vi "Load Plugin Management Core.vi"(11 "CIFPluginManager in":refnum<class "CIFPluginManager.lvclass">) -> (0 "error out":errorcluster)   [LabVIEW 2021, in "CIFPluginManager.lvclass"]
uses:
  CIFPluginManager.lvclass
  CIFPluginManager.lvclass/CIFPluginManager.ctl
  gRPC/CIF_Manager_server/RPC Service/Manager/Manager.lvclass
  C:/Program Files/National Instruments/LabVIEW 2021/vi.lib/gRPC/LabVIEW gRPC Servicer/ServiceBase/ServiceBase.lvclass
  gRPC/CIF_Manager_server/RPC Service/Manager/Manager.lvclass/Manager.ctl
  gRPC/CIF_Manager_server/RPC Messages/cif_manager_LoadPluginResponse.ctl
  gRPC/CIF_Manager_server/RPC Messages/cif_common_Status.ctl
  typedef/Plugin Load Command.ctl
  typedef/Loader Type.ctl
  CIFCore/Common/Typedef/Errors.ctl
  <vilib>/Utility/miscctls.llb/LVMapReplaceAction.ctl
  typedef/Loader Load Command.ctl
  gRPC/CIF_Manager_server/RPC Messages/cif_manager_AbortPluginResponse.ctl
  gRPC/CIF_Manager_server/RPC Messages/cif_manager_AbortAllPluginsResponse.ctl
  gRPC/CIF_Manager_server/RPC Messages/Get cif_manager_LoadPluginRequest.vi
  gRPC/CIF_Manager_server/RPC Messages/Set cif_manager_LoadPluginResponse.vi
  <vilib>/CIF Foundation/CIF Utilities/Errors/Append Error Location.vi
  gRPC/CIF_Manager_server/RPC Messages/Get cif_manager_AbortPluginRequest.vi
  gRPC/CIF_Manager_server/RPC Messages/Set cif_manager_AbortPluginResponse.vi
  gRPC/CIF_Manager_server/RPC Messages/Get cif_manager_AbortAllPluginsRequest.vi
  gRPC/CIF_Manager_server/RPC Messages/Set cif_manager_AbortAllPluginsResponse.vi
  gRPC/CIF_Manager_server/RPC Messages/Get cif_manager_LoadPluginRequest.vi/2ed25e12-861d-4677-8ead-ace2906b2041.vi
  gRPC/CIF_Manager_server/RPC Messages/FlatToRichcif_manager_LoadPluginRequest.vi
  gRPC/CIF_Manager_server/RPC Messages/Set cif_manager_LoadPluginResponse.vi/dcc74a39-081a-4bdd-860b-8ed792803c96.vi
  gRPC/CIF_Manager_server/RPC Messages/RichToFlatcif_manager_LoadPluginResponse.vi
  gRPC/CIF_Manager_server/RPC Messages/Get cif_manager_AbortPluginRequest.vi/2ed25e12-861d-4677-8ead-ace2906b2041.vi
  gRPC/CIF_Manager_server/RPC Messages/FlatToRichcif_manager_AbortPluginRequest.vi
  gRPC/CIF_Manager_server/RPC Messages/Set cif_manager_AbortPluginResponse.vi/dcc74a39-081a-4bdd-860b-8ed792803c96.vi
  gRPC/CIF_Manager_server/RPC Messages/RichToFlatcif_manager_AbortPluginResponse.vi
  gRPC/CIF_Manager_server/RPC Messages/Get cif_manager_AbortAllPluginsRequest.vi/2ed25e12-861d-4677-8ead-ace2906b2041.vi
  gRPC/CIF_Manager_server/RPC Messages/FlatToRichcif_manager_AbortAllPluginsRequest.vi
  gRPC/CIF_Manager_server/RPC Messages/Set cif_manager_AbortAllPluginsResponse.vi/dcc74a39-081a-4bdd-860b-8ed792803c96.vi
  gRPC/CIF_Manager_server/RPC Messages/RichToFlatcif_manager_AbortAllPluginsResponse.vi
  <vilib>/gRPC/LabVIEW gRPC Library/Shared/TranslateGrpcError.vi
  gRPC/CIF_Manager_server/RPC Messages/RichToFlatcif_common_Status.vi
  <vilib>/gRPC/LabVIEW gRPC Library/Server API/Server/Get Server DLL Path.vi
  <vilib>/Utility/error.llb/Error Cluster From Error Code.vi
  <vilib>/string/Create NI GUID.vi
  <vilib>/gRPC/LabVIEW gRPC Library/Server API/Message Requests/Complete Call.vi
  CIFUtilities/CIFLogs/CIFLogs.lvlib
  CIFCore/Common/CIFCoreCommon.lvlib
  CIFCore/Grpc/CIFCoreWrapper/CIFCoreWrapper.lvlib
  <vilib>/CIF Foundation/CIF Utilities/Time/Time_CIF_U.lvlib
  gRPC/CIF_Manager_Client_Wrapper/CIFManagerClientWrapper.lvlib
  CIFPluginLoader/gRPC/CIF_Plugin_Loader_Client_Wrapper/CIFPluginLoaderClientWrapper.lvlib
  gRPC/CIF_Manager_server/CIF_Manager_server.lvlib
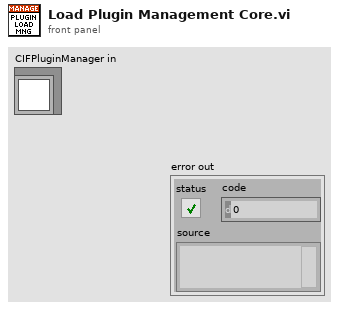
[diagram p1: front panel]
types:
  T1 = typedef "CIF_Manager_server.lvlib/Manager.lvclass/Server gRPC UEs.ctl" = cluster{"Manager LoadPlugin gRPC UE":refnum<user-event>, "Manager RegisterPlugin gRPC UE":refnum<user-event>, "Manager UnregisterPlugin gRPC UE":refnum<user-event>, "Manager QueryPluginTypes gRPC UE":refnum<user-event>, "Manager AbortPlugin gRPC UE":refnum<user-event>, "Manager UnloadAllPlugins gRPC UE":refnum<user-event>, "Manager Destroy gRPC UE":refnum<user-event>, "Manager Ping gRPC UE":refnum<user-event>, "Manager QueryErrors gRPC UE":refnum<user-event>, "Manager QueryConfig gRPC UE":refnum<user-event>, "Manager QueryInfo gRPC UE":refnum<user-event>, "Manager ResetErrorIndex gRPC UE":refnum<user-event>, "Manager ResetConfigIndex gRPC UE":refnum<user-event>, "Manager ResetInfoIndex gRPC UE":refnum<user-event>, "Manager QueryPluginInfo gRPC UE":refnum<user-event>, "Manager QueryPlugin gRPC UE":refnum<user-event>, "Manager QuerySystemStatus gRPC UE":refnum<user-event>, "Manager UpdateClock gRPC UE":refnum<user-event>, "Manager CreateOrch gRPC UE":refnum<user-event>, "Manager QueryClockStatus gRPC UE":refnum<user-event>, "Manager QueryAllChannels gRPC UE":refnum<user-event>, "Manager RegisterPluginLoader gRPC UE":refnum<user-event>, "Manager UnregisterPluginLoader gRPC UE":refnum<user-event>, "Manager CreatePluginLoader gRPC UE":refnum<user-event>, "Manager DestroyPluginLoader gRPC UE":refnum<user-event>, "Manager QueryPluginLoaders gRPC UE":refnum<user-event>}
  T2 = typedef "CIF_Manager_server.lvlib/cif_manager_LoadPluginResponse.ctl" = cluster{"status":T3}
  T3 = typedef "CIF_Manager_server.lvlib/cif_common_Status.ctl" = cluster{"code":i32, "message":string}
  T4 = typedef "CIFPluginManager.lvclass/Plugin Load Command.ctl" = cluster{"Plugin Name":string, "Plugin Path":string, "Loader Name":string, "Loader Type":T5}
  T5 = typedef "CIFPluginManager.lvclass/Loader Type.ctl" = enum16{"LabVIEW"}
  T6 = typedef "CIFCoreCommon.lvlib/Errors.ctl" = enum16{"Invalid Clock ID", "Long Sleep", "gRPC Server Not Found", "Config Parse", "Timestamp Wrap", "Delayed Execution", "Duplicate Channel", "Missing Channel", "Incorrect Type", "Flatten Error", "Unflatten Data", "Unique Name", "Plugin Not Found", "Plugin Type Not Found", "Plugin Version Not Found", "Manager Not Found", "Numerical Issue", "Time Jump", "Clock ID Match", "Channel Length", "Plugin Connection", "gRPC Server Connection", "PPL Name Match", "Build", "Config Log Parse", "Plugin Load", "UI Subpanel Load", "Python Name", "Invalid Name", "Unable to Change Ch Buffer", "Failed Kill", "Failed SysExec", "Function Not Implemented", "Load Timeout"}
  T7 = typedef "LVMapReplaceAction.ctl" = enum32{"Modify Entry only if found", "Add or Modify Entry", "Delete Entry"}
  T8 = typedef "CIFPluginManager.lvclass/Loader Load Command.ctl" = cluster{"Loader Type":T5, "Loader Name":string}
  T9 = typedef "CIF_Manager_server.lvlib/cif_manager_AbortPluginResponse.ctl" = cluster{"status":T3}
  T10 = typedef "CIF_Manager_server.lvlib/cif_manager_AbortAllPluginsResponse.ctl" = cluster{"status":T3}
  T11 = typedef "CIFPluginManager.lvclass/Plugin Management Data Map.ctl" = map{string, T12}
  T12 = typedef "CIFPluginManager.lvclass/Plugin Management Data.ctl" = cluster{"Unique Name":string, "Plugin Type":string, "gRPC Port":i32, "gRPC ID":T13, "Loader Type":T5, "Loader":string, "Version":T14, "Load Timestamp":i64, "Unload Timestamp":i64, "Unloading":bool, "Ready for removal":bool, "status":T15, "channels":T24}
  T13 = typedef "grpc-lvsupport-release.lvlib/grpcId.ctl" = u64
  T14 = typedef "CIFCoreCommon.lvlib/Version.ctl" = cluster{"Major":i32, "Minor":i32, "Fix":i32, "Build":i32}
  T15 = typedef "CIF_Manager_server.lvlib/cif_management_common_PluginStatusData.ctl" = cluster{"state":T16, "timing_statistics":T17, "fifo_statistics":T19, "error":T20, "monitor_doubles":T21, "monitor_u64s":T22, "monitor_i64s":T23}
  T16 = typedef "CIF_Manager_server.lvlib/cif_management_common_PluginStatusData_PluginState.ctl" = enum32{"PLUGINSTATE_UNKNOWN", "PLUGINSTATE_CREATING", "PLUGINSTATE_LISTENING", "PLUGINSTATE_RUNNING", "PLUGINSTATE_CLEANINGUP", "PLUGINSTATE_DESTROYING"}
  T17 = typedef "CIF_Manager_server.lvlib/cif_management_common_TimingStatistics.ctl" = cluster{"period":T18, "wake_error":T18, "execute":T18, "housekeep":T18, "idle":T18, "cleanup":T18, "custom_1":T18, "custom_2":T18}
  T18 = typedef "CIF_Manager_server.lvlib/cif_common_TimingStats.ctl" = cluster{"max":i64, "min":i64, "avg":dbl}
  T19 = typedef "CIF_Manager_server.lvlib/cif_management_common_FifoStatistics.ctl" = cluster{"from_t0":T18, "from_previous_plugin":T18, "output_error":T18}
  T20 = typedef "CIF_Manager_server.lvlib/cif_management_common_Error.ctl" = cluster{"status":bool, "code":i32}
  T21 = typedef "CIF_Manager_server.lvlib/cif_management_common_MonitorDoubles.ctl" = cluster{"double_1":dbl, "double_2":dbl, "double_3":dbl, "double_4":dbl}
  T22 = typedef "CIF_Manager_server.lvlib/cif_management_common_MonitorU64.ctl" = cluster{"u64_1":u64, "u64_2":u64, "u64_3":u64, "u64_4":u64}
  T23 = typedef "CIF_Manager_server.lvlib/cif_management_common_MonitorI64.ctl" = cluster{"i64_1":i64, "i64_2":i64, "i64_3":i64, "i64_4":i64}
  T24 = typedef "CIF_Manager_server.lvlib/cif_management_common_Channels.ctl" = cluster{"channels":T25[]}
  T25 = typedef "CIF_Manager_server.lvlib/cif_management_common_Channel.ctl" = cluster{"name":string, "direction":T26, "type":string, "custom_config":u8[], "connected":bool, "connected_name":string, "forced":bool, "channel_pattern":T27}
  T26 = typedef "CIF_Manager_server.lvlib/cif_management_common_ChannelDirection.ctl" = enum32{"CHANNELDIRECTION_UNKNOWN", "CHANNELDIRECTION_PUBLISHER", "CHANNELDIRECTION_SUBSCRIBER"}
  T27 = typedef "CIF_Manager_server.lvlib/cif_management_common_ChannelPattern.ctl" = enum32{"CHANNELPATTERN_UNKNOWN", "CHANNELPATTERN_TAG", "CHANNELPATTERN_FIFO", "CHANNELPATTERN_MULTIFIFO", "CHANNELPATTERN_BACKPRESSUREFIFO"}
  T28 = typedef "CIF_Manager_server.lvlib/cif_manager_LoadPluginRequest.ctl" = cluster{"plugin_type":string, "plugin_name":string, "version":string, "loader_process":string}
  T29 = typedef "CIFPluginManager.lvclass/Discovered Plugin.ctl" = cluster{"Filename":string, "Plugin Type":string, "Qualified name":string, "Version":T14, "Plugin Metadata":T30, "Loader Type":T5, "File Path":string, "Relative Path":string[]}
  T30 = typedef "CIFPluginManager.lvclass/Plugin Metadata.ctl" = cluster{"Description":string, "History":string, "Author":string}
  T31 = typedef "CIF_Manager_client.lvlib/cif_common_Status.ctl" = cluster{"code":i32, "message":string}
  T32 = typedef "CIFPluginManager.lvclass/Loader Map.ctl" = map{string, T33}
  T33 = typedef "CIFPluginManager.lvclass/Loaders.ctl" = cluster{"Loader Type":T5, "grpc_port":i32, "pid":u32, "gRPC ID":T13, "Load Timestamp":i64, "Unloading":bool, "Ready for removal":bool, "Unload Timestamp":i64}
  T34 = typedef "CIF_Manager_server.lvlib/cif_manager_AbortPluginRequest.ctl" = cluster{"plugin_name":string}
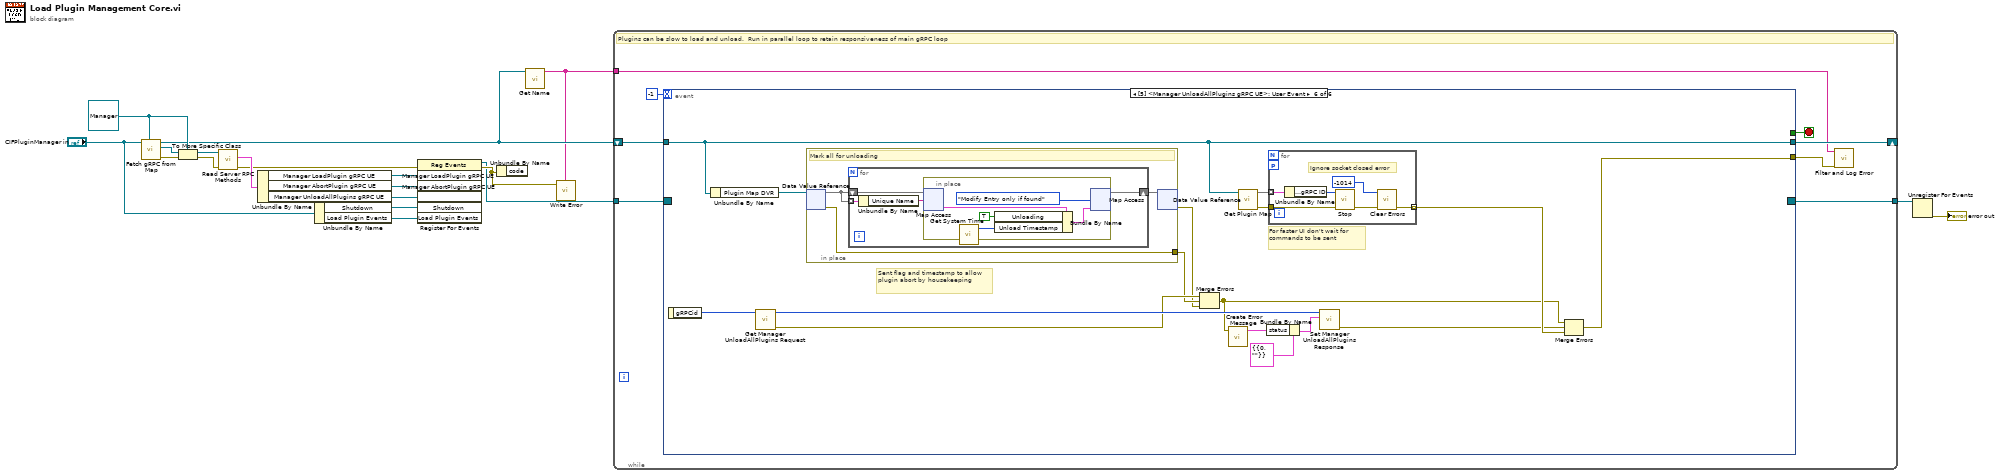
[diagram p0: block diagram]
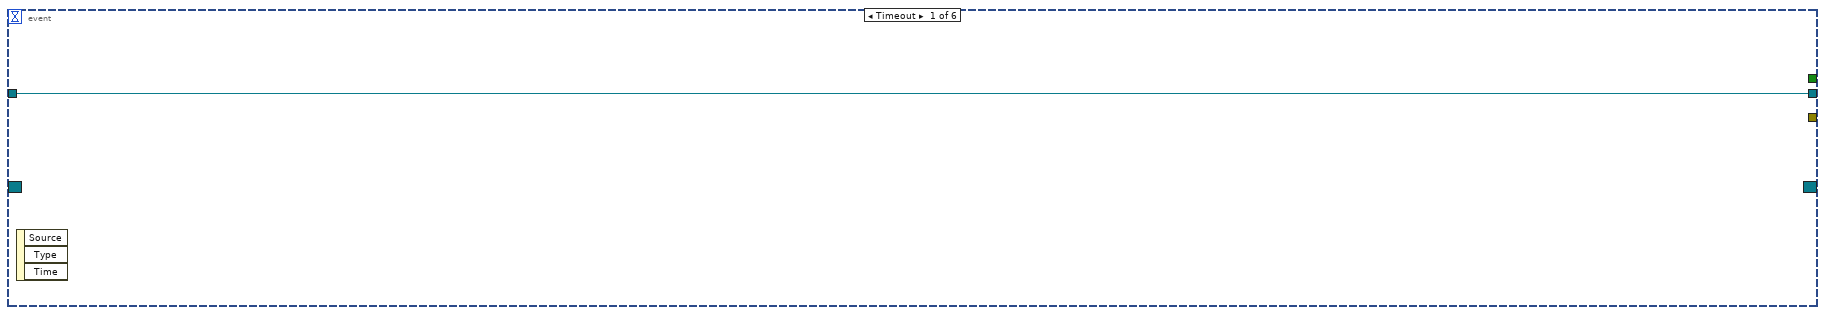
[diagram p2: hidden frame]
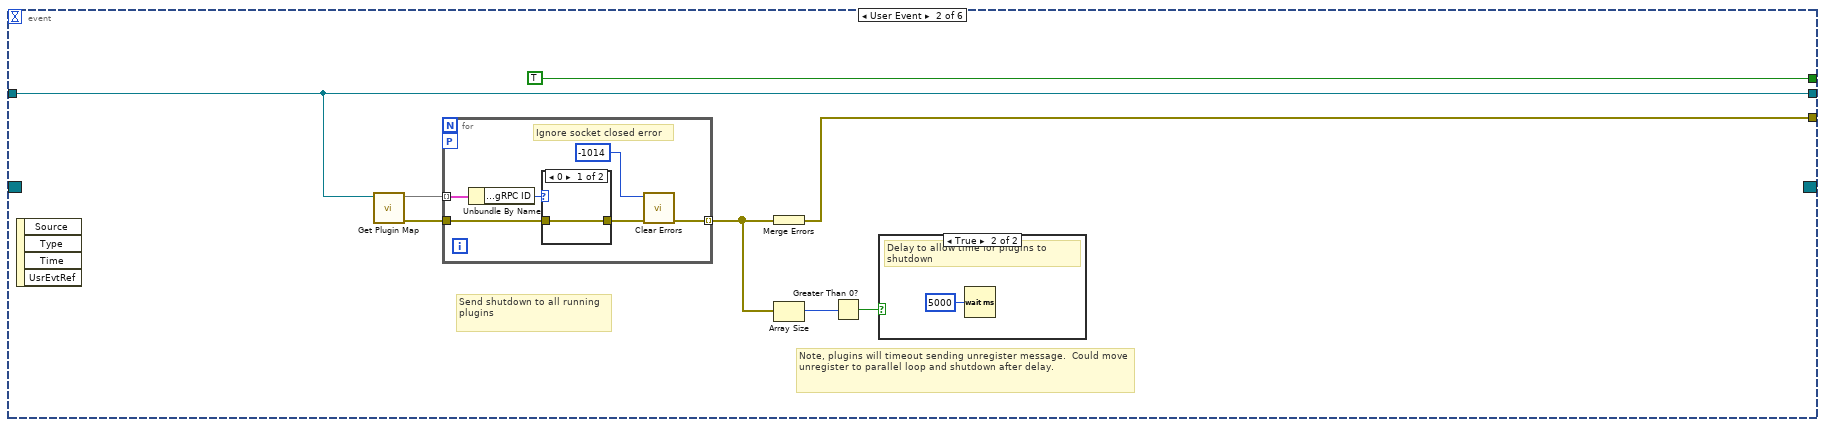
[diagram p3: hidden frame]
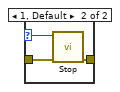
[diagram p5: hidden frame]
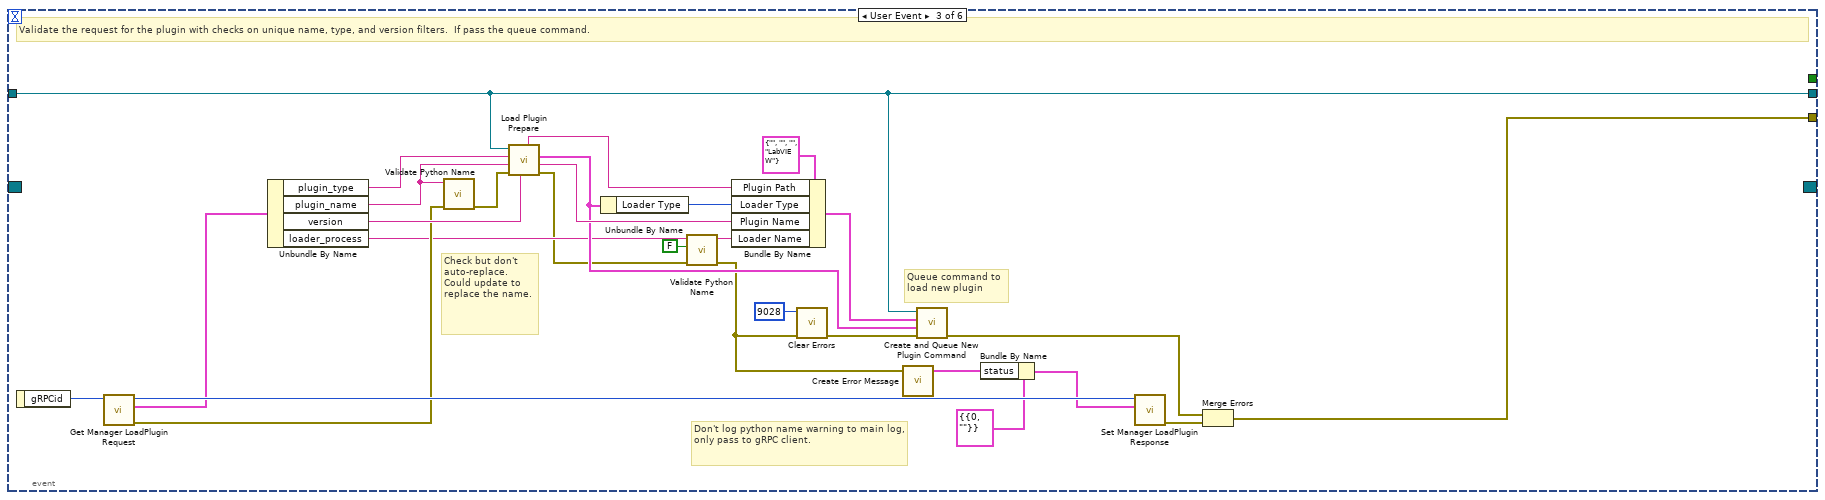
[diagram p6: hidden frame]
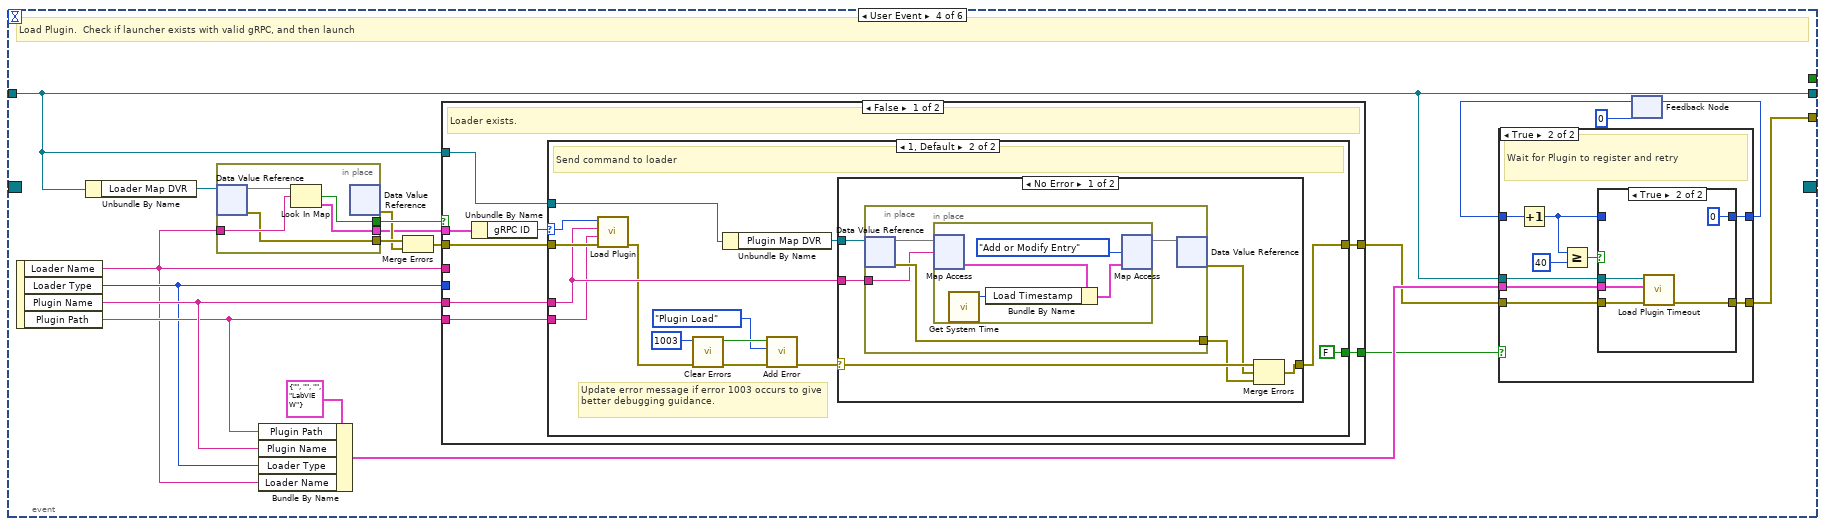
[diagram p7: hidden frame]
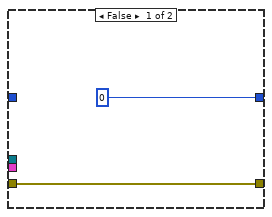
[diagram p8: hidden frame]
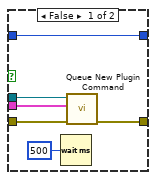
[diagram p9: hidden frame]
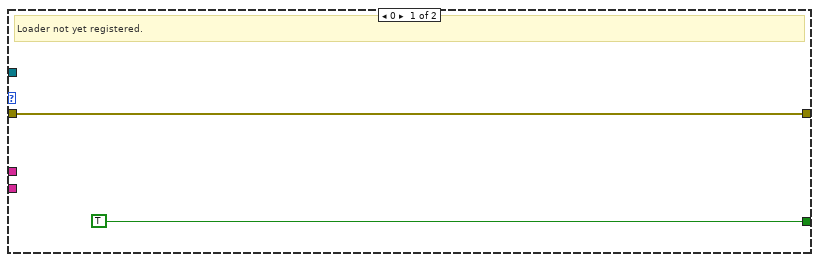
[diagram p10: hidden frame]
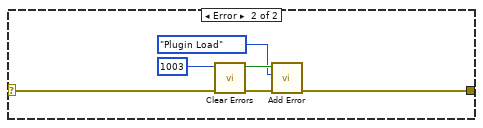
[diagram p11: hidden frame]
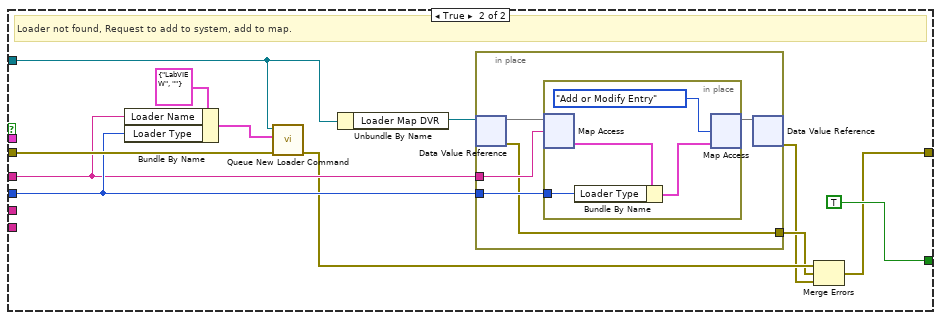
[diagram p12: hidden frame]
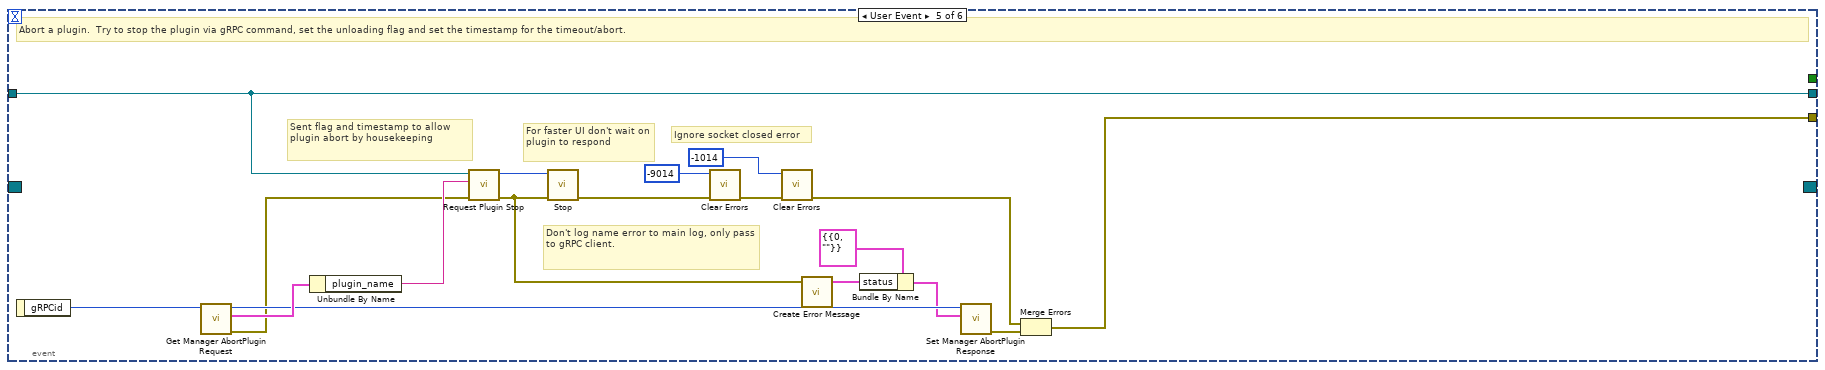
[diagram p13: hidden frame]
diagram:
  w16 = refnum<class "Manager.lvclass"> refnum ("CIF_Manager_server.lvlib:Manager.lvclass")
  n1 = call "Fetch gRPC from Map.vi"("gRPC Server Class type"=w16, "Plugin Manager in"="CIFPluginManager in") -> ("error out"=w15:errorcluster, "gRPC Server Class out"=w17:refnum<class "ServiceBase.lvclass">, "Plugin Manager out"=w2:refnum<class "CIFPluginManager.lvclass">)  [unwired: 7 in]
  n2 = To More Specific Class(target class=w16, reference=w17, error in=w15) -> (specific class reference=w13:refnum<class "Manager.lvclass">, error out=w14:errorcluster)
  n3 = call "Read Server RPC Methods.vi"("error in (no error)"=w14, "gRPC service in"=w13) -> ("error out"=w8:errorcluster, "Server RPC Methods"=w9:T1)  [unwired: 7 in, 1 out]
  n4 = Unbundle By Name(w9) -> ("Manager LoadPlugin gRPC UE"=w4:refnum<user-event>, "Manager AbortPlugin gRPC UE"=w5:refnum<user-event>, "Manager UnloadAllPlugins gRPC UE"=w6:refnum<user-event>)
  n5 = Unbundle By Name("CIFPluginManager in") -> ("Shutdown"=w7:refnum<user-event>, "Load Plugin Events"=w3:refnum<user-event>)
  n6 = register-events(error in=w8, w4, w5, w6, w7, w3) -> (reference out=w10:refnum<event-registration>, error out=w11:errorcluster)  [unwired: 1 in]
  n7 = Unbundle By Name(w11) -> ()  [unwired: 1 out]
  n8 = call "Get Name.vi"("CIFPluginManager in"=w2) -> ("Name"=w1:string)  [unwired: 10 in]
  n9 = call "Write Error.vi"("error in (no error)"=w11, "Plugin Name"=w1) -> ()  [unwired: 2 in, 1 out]
  n10 = while {
    tunnel: w10 -> [w21]
    shift-right: [w23] -> _
    shift-left: w2 -> [w27]
    tunnel: [w24] -> w18
    tunnel: w1 -> [w20]
    stop <- w25 stop-if-true
    # "Plugins can be slow to load and unload.  Run in parallel loop to retain responsiveness of main gRPC loop"
    n11 = event shown="[5] <Manager UnloadAllPlugins gRPC UE>: User Event" {
      selector: w21 -> [_ _ _ _ _ _]
      dyn-events: [_ _ _ _ _ _] -> w24
      timeout: -1 -> [_ _ _ _ _ _]
      tunnel: w27 -> [w28 w34 w59 w80 w197 w214]
      tunnel: [w28 w34 w59 w80 w197 w214] -> w23
      tunnel: [_ TRUE _ _ _ _] -> w25
      tunnel: [_ w33 w68 w76 w199 w211] -> w22
      event Timeout {
        n12 = event-data() -> ()  [unwired: 1 in, 3 out]
      }
      event User Event {
        # "Note, plugins will timeout sending unregister message.  Could move unregister to parallel loop and shutdown after delay."
        # "Send shutdown to all running plugins"
        n13 = event-data() -> ()  [unwired: 1 in, 4 out]
        n14 = call "Get Plugin Map.vi"("CIFPluginManager in"=w34) -> ("error out"=w35:errorcluster, "Plugin Map"=w32:T11)  [unwired: 9 in]
        n15 = for {
          tunnel: w35 -> [w42]
          tunnel: w32 -> [w43] mode=indexing
          workers-P: _ -> [_]
          tunnel: [w39] -> w31 mode=indexing
          # "Ignore socket closed error"
          n16 = Unbundle By Name(w43) -> ("Plugin Management Data.gRPC ID"=w38:T13)
          n17 = case shown="0" w38 {
            selector: w38 -> [_ w45]
            tunnel: w42 -> [w44 w47]
            tunnel: [w44 w46] -> w40
            frame 0 {
            }
            frame 1, Default {
              n18 = call "Stop.vi"("error in"=w47, "gRPC ID"=w45) -> ("error out"=w46:errorcluster)  [unwired: 8 in, 1 out]
            }
          }
          n19 = call <vilib>:"Clear Errors.vi"("error in (no error)"=w40, "specific error code to clear (0: all)"=-1014) -> ("error out"=w39:errorcluster)  [unwired: 4 in, 1 out]
        }
        n20 = Merge Errors(w31) -> (w33:errorcluster)
        n21 = Array Size(array=w31) -> (size(s)=w30:i32)
        n22 = Greater Than 0?(x=w30) -> (x > 0?=w29:bool)
        n23 = case shown="True" w29 {
          frame False {
          }
          frame True {
            # "Delay to allow time for plugins to shutdown"
            n24 = Wait (ms)(milliseconds to wait=u32 5000) -> ()  [unwired: 1 out]
          }
        }
      }
      event User Event {
        # "Queue command to load new plugin"
        # "Don't log python name warning to main log, only pass to gRPC client."
        # "Check but don't auto-replace.  Could update to replace the name."
        # "Validate the request for the plugin with checks on unique name, type, and version filters.  If pass the queue command."
        n25 = event-data() -> ("gRPCid"=w67:T13)  [unwired: 1 in]
        n26 = call "Get Manager LoadPlugin Request.vi"("gRPCid"=w67) -> ("error out"=w69:errorcluster, "Message Data"=w73:T28, "gRPCid out"=w75:T13)  [unwired: 8 in]
        n27 = Unbundle By Name(w73) -> ("plugin_type"=w56:string, "plugin_name"=w70:string, "version"=w72:string, "loader_process"=w55:string)
        n28 = call "Validate Python Name.vi"("error in (no error)"=w69, "Name In"=w70) -> ("error out"=w71:errorcluster)  [unwired: 8 in, 1 out]
        n29 = call "Load Plugin Prepare.vi"("Version String"=w72, "error in (no error)"=w71, "Unique Name"=w70, "Plugin Type"=w56, "CIFPluginManager in"=w59) -> ("error out"=w52:errorcluster, "Unique Name (dup)"=w60:string, "Matching Plugin"=w58:T29, "path"=w62:string)  [unwired: 3 in]
        n30 = Unbundle By Name(w58) -> ("Loader Type"=w61:T5)
        n31 = call "Validate Python Name.vi"("error in (no error)"=w52, "GUID for Empty"=FALSE, "Name In"=w55) -> ("error out"=w51:errorcluster, "Valid Name"=w54:string)  [unwired: 7 in]
        n32 = Bundle By Name(cluster=T4 {"Plugin Name"="", "Plugin Path"="", "Loader Name"="", "Loader Type"=enum."LabVIEW"} ("New Plugin"), "Plugin Path"=w62, "Loader Type"=w61, "Plugin Name"=w60, "Loader Name"=w54) -> (w64:T4)
        n33 = call <vilib>:"Clear Errors.vi"("error in (no error)"=w51, "specific error code to clear (0: all)"=9028) -> ("error out"=w65:errorcluster)  [unwired: 4 in, 1 out]
        n34 = call "Create Error Message.vi"("error in (no error)"=w51) -> ("Error Message"=w49:T31)  [unwired: 3 in]
        n35 = call "Create and Queue New Plugin Command.vi"("error in (no error)"=w65, "Matching Plugin"=w58, "New Plugin"=w64, "CIFPluginManager in"=w59) -> ("error out"=w57:errorcluster)  [unwired: 7 in]
        n36 = Bundle By Name(cluster=T2 {"status"={"code"=0, "message"=""}} ("Message Data"), "status"=w49) -> (w48:T2)
        n37 = call "Set Manager LoadPlugin Response.vi"("Message Data"=w48, "gRPCid in"=w75) -> ("error out"=w74:errorcluster)  [unwired: 9 in]
        n38 = Merge Errors(w57, w74) -> (w68:errorcluster)
      }
      event User Event {
        # "Load Plugin.  Check if launcher exists with valid gRPC, and then launch"
        n39 = event-data() -> ("Loader Name"=w84:string, "Loader Type"=w85:T5, "Plugin Name"=w87:string, "Plugin Path"=w86:string)  [unwired: 1 in]
        n40 = Unbundle By Name(w80) -> ("Loader Map DVR"=w94:refnum<data-value>)
        n41 = in-place {
          in-place-border: w84 -> [w185]
          in-place-border: [w184] -> w92
          in-place-border: [w183] -> w89
          in-place-border: [w182] -> w93
          n42 = in-place-dvr #1(w94) -> (w186:T32, w184:errorcluster)
          n43 = Look In Map(map=w186, key=w185) -> (key not found?=w182:bool, value=w183:T33)  [unwired: 1 in]
          n44 = in-place-dvr #1() -> (w91:errorcluster)  [unwired: 1 in, 1 out]
        }
        n45 = Bundle By Name(cluster=T4 {"Plugin Name"="", "Plugin Path"="", "Loader Name"="", "Loader Type"=enum."LabVIEW"} ("New Plugin"), "Plugin Path"=w86, "Plugin Name"=w87, "Loader Type"=w85, "Loader Name"=w84) -> (w79:T4)
        n46 = Merge Errors(w92, w91) -> (w90:errorcluster)
        n47 = case shown="False" w93 {
          tunnel: w80 -> [w117 w168]
          tunnel: w90 -> [w118 w172]
          tunnel: [w119 w161] -> w78
          tunnel: w85 -> [_ w166]
          tunnel: w84 -> [_ w165]
          tunnel: [w122 TRUE] -> w77
          tunnel: w89 -> [w124 _]
          tunnel: w87 -> [w121 _]
          tunnel: w86 -> [w120 _]
          frame False {
            # "Loader exists."
            n48 = Unbundle By Name(w124) -> ("gRPC ID"=w123:T13)
            n49 = case shown="1, Default" w123 {
              selector: w123 -> [_ w140]
              tunnel: [TRUE FALSE] -> w122
              tunnel: w121 -> [_ w136]
              tunnel: w120 -> [_ w135]
              tunnel: [w125 w137] -> w119
              tunnel: w118 -> [w125 w139]
              tunnel: w117 -> [_ w134]
              frame 0 {
                # "Loader not yet registered."
              }
              frame 1, Default {
                # "Update error message if error 1003 occurs to give better debugging guidance."
                # "Send command to loader"
                n50 = call "Load Plugin.vi"("error in"=w139, "Plugin Path"=w135, "Plugin Name"=w136, "gRPC ID in"=w140) -> ("error out"=w129:errorcluster)  [unwired: 6 in, 1 out]
                n51 = call <vilib>:"Clear Errors.vi"("error in (no error)"=w129, "specific error code to clear (0: all)"=1003) -> ("error out"=w132:errorcluster, "specific error cleared?"=w131:bool)  [unwired: 4 in]
                n52 = Unbundle By Name(w134) -> ("Plugin Map DVR"=w133:refnum<data-value>)
                n53 = call "Add Error.vi"("error in (no error)"=w132, "Error"=Errors."Plugin Load", "Insert Error"=w131) -> ("error out"=w128:errorcluster)  [unwired: 8 in]
                n54 = case shown="No Error" w128 {
                  selector: w128 -> [w145 w156]
                  tunnel: w136 -> [w146 _]
                  tunnel: [w142 w155] -> w137
                  tunnel: w133 -> [w141 _]
                  frame No Error {
                    n55 = in-place {
                      in-place-border: w146 -> [w148]
                      in-place-border: [w150] -> w144
                      n56 = in-place-dvr #2(w141) -> (w149:T11, w150:errorcluster)
                      n57 = in-place {
                        n58 = in-place-map #3(w149, w148) -> (w154:T12)  [unwired: 1 in, 1 out]
                        n59 = call <vilib>:"Get System Time.vi"() -> ("Time (ns)"=w151:i64)  [unwired: 5 in]
                        n60 = Bundle By Name(cluster=w154, "Load Timestamp"=w151) -> (w153:T12)
                        n61 = in-place-map #3(w153, LVMapReplaceAction."Add or Modify Entry" ("action")) -> (w147:T11)  [unwired: 2 out]
                      }
                      n62 = in-place-dvr #2(w147) -> (w143:errorcluster)  [unwired: 1 out]
                    }
                    n63 = Merge Errors(w145, w143, w144) -> (w142:errorcluster)
                  }
                  frame Error {
                    n64 = call <vilib>:"Clear Errors.vi"("error in (no error)"=w156, "specific error code to clear (0: all)"=1003) -> ("error out"=w160:errorcluster, "specific error cleared?"=w159:bool)  [unwired: 4 in]
                    n65 = call "Add Error.vi"("error in (no error)"=w160, "Error"=Errors."Plugin Load", "Insert Error"=w159) -> ("error out"=w155:errorcluster)  [unwired: 8 in]
                  }
                }
              }
            }
          }
          frame True {
            # "Loader not found, Request to add to system, add to map."
            n66 = Bundle By Name(cluster=T8 {"Loader Type"=enum."LabVIEW", "Loader Name"=""} ("New Launcher"), "Loader Name"=w165, "Loader Type"=w166) -> (w170:T8)
            n67 = call "Queue New Loader Command.vi"("error in (no error)"=w172, "New Launcher"=w170, "CIFPluginManager in"=w168) -> ("error out"=w164:errorcluster)  [unwired: 8 in]
            n68 = Unbundle By Name(w168) -> ("Loader Map DVR"=w167:refnum<data-value>)
            n69 = in-place {
              in-place-border: w166 -> [w175]
              in-place-border: w165 -> [w174]
              in-place-border: [w173] -> w163
              n70 = in-place-dvr #4(w167) -> (w177:T32, w173:errorcluster)
              n71 = in-place {
                in-place-border: w175 -> [w178]
                n72 = in-place-map #5(w177, w174) -> (w180:T33)  [unwired: 1 in, 1 out]
                n73 = Bundle By Name(cluster=w180, "Loader Type"=w178) -> (w179:T33)
                n74 = in-place-map #5(w179, LVMapReplaceAction."Add or Modify Entry" ("action")) -> (w176:T32)  [unwired: 2 out]
              }
              n75 = in-place-dvr #4(w176) -> (w162:errorcluster)  [unwired: 1 out]
            }
            n76 = Merge Errors(w164, w163, w162) -> (w161:errorcluster)
          }
        }
        n77 = feedback #6(0) -> (w83:i32)
        n78 = case shown="True" w77 {
          tunnel: w78 -> [w96 w103]
          tunnel: w80 -> [_ w105]
          tunnel: w79 -> [_ w104]
          tunnel: [w96 w102] -> w76
          tunnel: w83 -> [_ w101]
          tunnel: [0 w97] -> w81
          frame False {
          }
          frame True {
            # "Wait for Plugin to register and retry"
            n79 = Increment(x=w101) -> (x+1=w98:i32)
            n80 = Greater Or Equal?(x=w98, y=40) -> (x >= y?=w100:bool)
            n81 = case shown="True" w100 {
              tunnel: w105 -> [w108 w112]
              tunnel: w104 -> [w107 w113]
              tunnel: w103 -> [w110 w115]
              tunnel: [w109 w114] -> w102
              tunnel: w98 -> [w106 _]
              tunnel: [w106 0] -> w97
              frame False {
                n82 = Wait (ms)(milliseconds to wait=u32 500) -> ()  [unwired: 1 out]
                n83 = call "Queue New Plugin Command.vi"("error in (no error)"=w110, "New Plugin"=w107, "CIFPluginManager in"=w108) -> ("error out"=w109:errorcluster)  [unwired: 8 in]
              }
              frame True {
                n84 = call "Load Plugin Timeout.vi"("error in (no error)"=w115, "New Plugin"=w113, "CIFPluginManager in"=w112) -> ("error out"=w114:errorcluster)  [unwired: 8 in]
              }
            }
          }
        }
        n85 = feedback-in #6(w81) -> ()
      }
      event User Event {
        # "Sent flag and timestamp to allow plugin abort by housekeeping"
        # "Ignore socket closed error"
        # "Don't log name error to main log, only pass to gRPC client."
        # "For faster UI don't wait on plugin to respond"
        # "Abort a plugin.  Try to stop the plugin via gRPC command, set the unloading flag and set the timestamp for the timeout/abort."
        n86 = event-data() -> ("gRPCid"=w200:T13)  [unwired: 1 in]
        n87 = call "Get Manager AbortPlugin Request.vi"("gRPCid"=w200) -> ("error out"=w198:errorcluster, "Message Data"=w203:T34, "gRPCid out"=w201:T13)  [unwired: 8 in]
        n88 = Unbundle By Name(w203) -> ("plugin_name"=w204:string)
        n89 = call "Request Plugin Stop.vi"("error in (no error)"=w198, "Unique Name"=w204, "CIFPluginManager in"=w197) -> ("error out"=w195:errorcluster, "gRPC ID"=w196:T13)  [unwired: 7 in]
        n90 = call "Stop.vi"("error in"=w195, "gRPC ID"=w196) -> ("error out"=w193:errorcluster)  [unwired: 8 in, 1 out]
        n91 = call <vilib>:"Clear Errors.vi"("error in (no error)"=w193, "specific error code to clear (0: all)"=-9014) -> ("error out"=w191:errorcluster)  [unwired: 4 in, 1 out]
        n92 = call <vilib>:"Clear Errors.vi"("error in (no error)"=w191, "specific error code to clear (0: all)"=-1014) -> ("error out"=w190:errorcluster)  [unwired: 4 in, 1 out]
        n93 = call "Create Error Message.vi"("error in (no error)"=w195) -> ("Error Message"=w188:T31)  [unwired: 3 in]
        n94 = Bundle By Name(cluster=T9 {"status"={"code"=0, "message"=""}} ("Message Data"), "status"=w188) -> (w187:T9)
        n95 = call "Set Manager AbortPlugin Response.vi"("Message Data"=w187, "gRPCid in"=w201) -> ("error out"=w202:errorcluster)  [unwired: 9 in]
        n96 = Merge Errors(w190, w202) -> (w199:errorcluster)
      }
      event User Event {
        # "Sent flag and timestamp to allow plugin abort by housekeeping"
        # "For faster UI don't wait for commands to be sent"
        n97 = event-data() -> ("gRPCid"=w219:T13)  [unwired: 1 in]
        n98 = Unbundle By Name(w214) -> ("Plugin Map DVR"=w220:refnum<data-value>)
        n99 = call "Get Manager UnloadAllPlugins Request.vi"("gRPCid"=w219) -> ("error out"=w217:errorcluster, "gRPCid out"=w218:T13)  [unwired: 8 in, 1 out]
        n100 = in-place {
          in-place-border: [w227] -> w216
          # "Mark all for unloading"
          n101 = in-place-dvr #7(w220) -> (w229:T11, w227:errorcluster)
          n102 = for {
            tunnel: w229 -> [w231] mode=indexing
            shift-right: [w232] -> w228
            shift-left: w229 -> [w233]
            n103 = Unbundle By Name(w231) -> ("Unique Name"=w230:string)
            n104 = in-place {
              n105 = in-place-map #8(w233, w230) -> (w235:T12)  [unwired: 1 in, 1 out]
              n106 = call <vilib>:"Get System Time.vi"() -> ("Time (ns)"=w236:i64)  [unwired: 5 in]
              n107 = Bundle By Name(cluster=w235, "Unloading"=TRUE, "Unload Timestamp"=w236) -> (w234:T12)
              n108 = in-place-map #8(w234, LVMapReplaceAction."Modify Entry only if found" ("action")) -> (w232:T11)  [unwired: 2 out]
            }
          }
          n109 = in-place-dvr #7(w228) -> (w215:errorcluster)  [unwired: 1 out]
        }
        n110 = Merge Errors(w217, w216, w215) -> (w209:errorcluster)
        n111 = call "Create Error Message.vi"("error in (no error)"=w209) -> ("Error Message"=w206:T31)  [unwired: 3 in]
        n112 = call "Get Plugin Map.vi"("CIFPluginManager in"=w214) -> ("error out"=w212:errorcluster, "Plugin Map"=w213:T11)  [unwired: 9 in]
        n113 = Bundle By Name(cluster=T10 {"status"={"code"=0, "message"=""}} ("Message Data"), "status"=w206) -> (w205:T10)
        n114 = for {
          tunnel: w212 -> [w224]
          tunnel: w213 -> [w225] mode=indexing
          workers-P: _ -> [_]
          tunnel: [w222] -> w210 mode=indexing
          # "Ignore socket closed error"
          n115 = Unbundle By Name(w225) -> ("Plugin Management Data.gRPC ID"=w226:T13)
          n116 = call "Stop.vi"("error in"=w224, "gRPC ID"=w226) -> ("error out"=w223:errorcluster)  [unwired: 8 in, 1 out]
          n117 = call <vilib>:"Clear Errors.vi"("error in (no error)"=w223, "specific error code to clear (0: all)"=-1014) -> ("error out"=w222:errorcluster)  [unwired: 4 in, 1 out]
        }
        n118 = call "Set Manager UnloadAllPlugins Response.vi"("Message Data"=w205, "gRPCid in"=w218) -> ("error out"=w208:errorcluster)  [unwired: 9 in]
        n119 = Merge Errors(w209, w208, w210) -> (w211:errorcluster)
      }
    }
    n120 = call "Filter and Log Error.vi"("error In"=w22, "Name"=w20) -> ()  [unwired: 10 in]
  }
  n121 = Unregister For Events(event registration refnum=w18) -> (error out=→"error out":errorcluster)  [unwired: 1 in]
